vi "Import Project Information From Excel.vi"(0 "Project  path":path=path "C:/Users/L025200.LUXSHARE/Desktop/VNA Aotomatic Data Save Tool 20150327/Project/QSFP+ Project.xls" caption="Project path") -> (16 "Switch Matrix  Name":string, 17 "Report Config":string[](array[string]), 18 "Spec Name":string, 19 "Report Name":string, 20 "S-para Pair Name":string[](array[string])=["TX0", "TX1", "TX2", "TX3", "RX0", "RX1", "RX2", "RX3"], 22 "NEXT Pair Name":string[](array[string])=["TX0-RX0", "TX1-RX0", "TX2-RX0", "TX3-RX0", "TX0-RX1", "TX1-RX1", "TX2-RX1", "TX3-RX1", "TX0-RX2", "TX1-RX2", "TX2-RX2", "TX3-RX2", "TX0-RX3", "TX1-RX3", "TX2-RX3", "TX3-RX3"], 23 "SingleTest Item Name":string[](array[string]), 24 "FEXT Pair Name":string[](array[string])=["TX1-RX0", "TX2-RX0", "TX3-RX0", "TX0-RX1", "TX2-RX1", "TX3-RX1", "TX0-RX2", "TX1-RX2", "TX3-RX2", "TX0-RX3", "TX1-RX3", "TX2-RX3"], 25 "Diff Test Item Name":string[](array[string])=["SDD21", "SDD22", "SCD21", "SCD22", "SCC11", "SCC22", "NEXT", "FEXT"], 26 "Spec Association Col No":string[](array[string])=["1", "2", "NAN", "NAN", "NAN", "NAN", "NAN", "NAN"], 27 "Cal File Path":string[](array[string])=["D:\\CALFILES\\cable.csa"])   [LabVIEW 2011]
panel:
  in  "Excel._Worksheet":refnum<k7>
  in  "Excel._Application":refnum<k7>
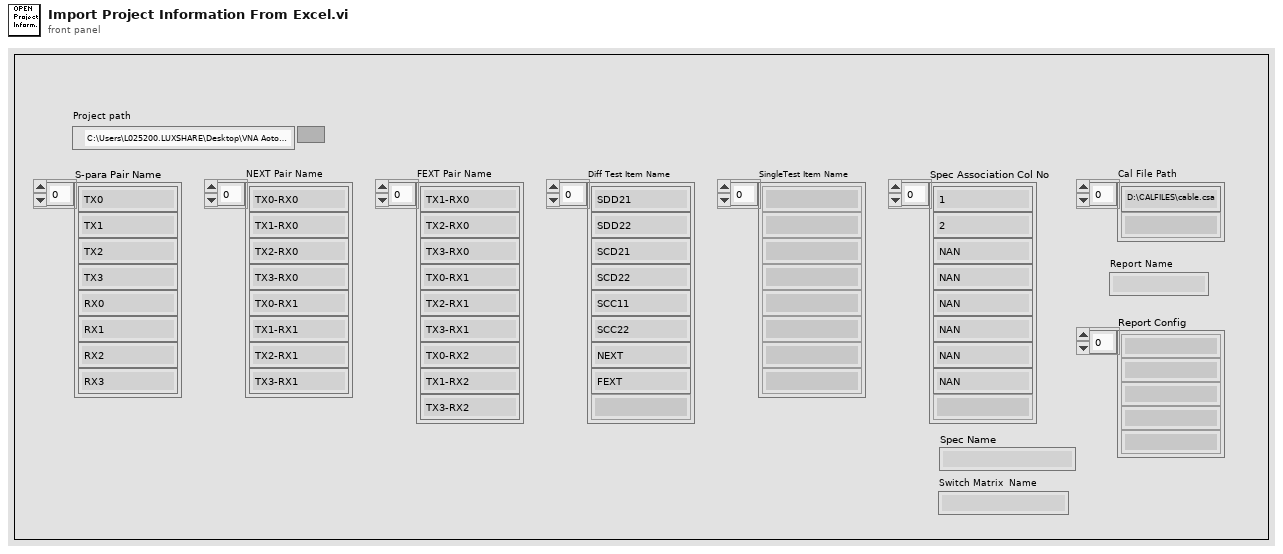
[diagram p1: front panel]
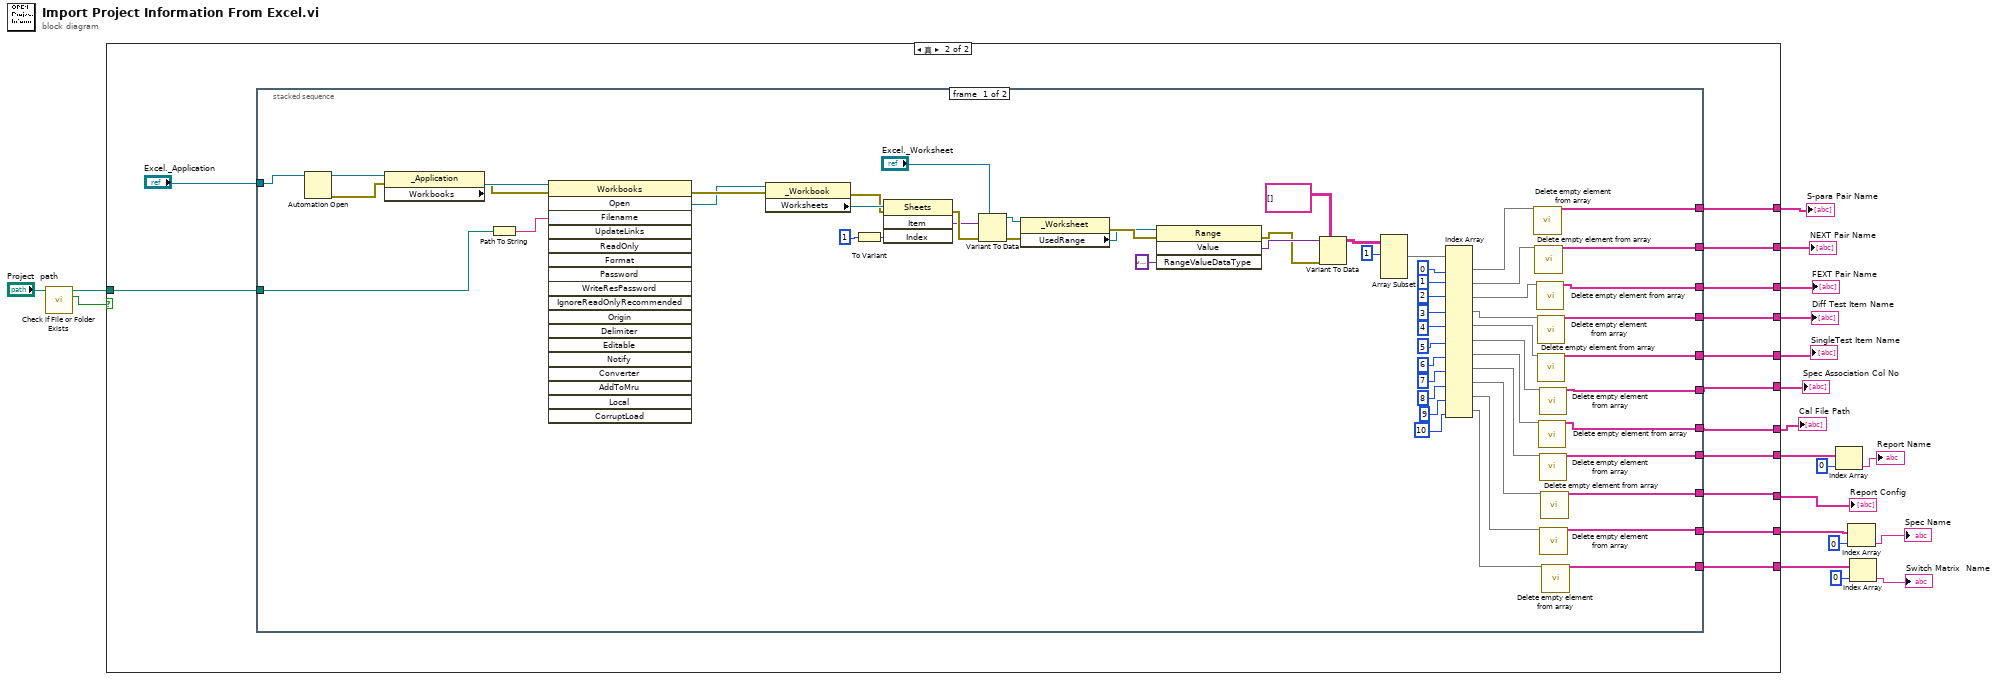
[diagram p0: block diagram]
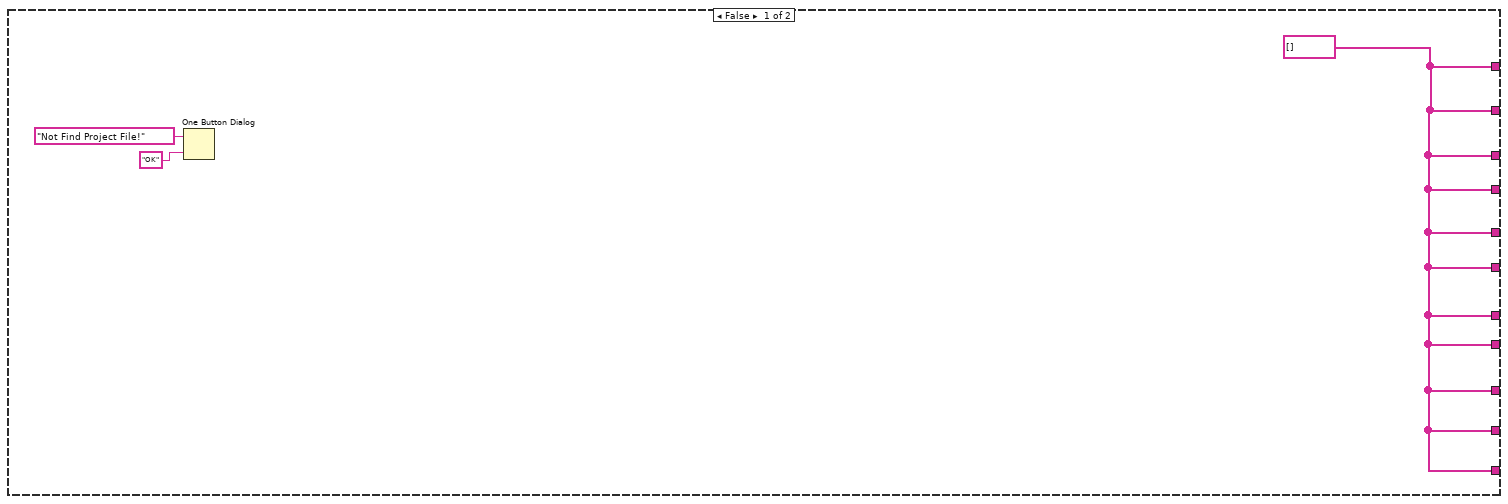
[diagram p2: hidden frame]
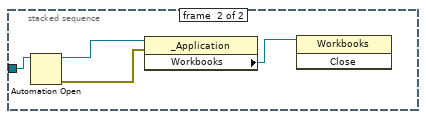
[diagram p3: hidden frame]
diagram:
  n1 = call <vilib>:"Check if File or Folder Exists.vi"("path"="Project  path") -> ("file or folder exists?"=w20:bool, "dup path"=w19:path)  [unwired: 8 in, 1 out]
  n2 = case shown="真" w20 {
    tunnel: w19 -> [_ w35]
    tunnel: [w21 w34] -> w18
    tunnel: [w21 w33] -> w17
    tunnel: [w21 w32] -> w16
    tunnel: [w21 w31] -> w15
    tunnel: [w21 w30] -> w14
    tunnel: [w21 w29] -> w12
    tunnel: [w21 w28] -> w11
    tunnel: [w21 w27] -> w10
    tunnel: [w21 w26] -> w7
    tunnel: [w21 w25] -> w4
    tunnel: [w21 w24] -> w3
    frame False {
      w21 = string[] []
      n3 = One Button Dialog(message="Not Find Project File!" ("消息"), button name ("OK")="OK" ("按钮名称（“确定”）")) -> ()  [unwired: 1 out]
    }
    frame True {
      n4 = stacked-sequence {
        tunnel: "Excel._Application" -> [w61 w98]
        tunnel: w35 -> [w69 _]
        tunnel: [w67 _] -> w34
        tunnel: [w66 _] -> w33
        tunnel: [w65 _] -> w32
        tunnel: [w56 _] -> w30
        tunnel: [w50 _] -> w31
        tunnel: [w51 _] -> w29
        tunnel: [w49 _] -> w28
        tunnel: [w44 _] -> w27
        tunnel: [w43 _] -> w26
        tunnel: [w38 _] -> w25
        tunnel: [w37 _] -> w24
        frame #0 {
          n5 = Automation Open(Automation Refnum=w61) -> (Automation Refnum=w62:refnum<k7>, error out=w96:errorcluster)  [unwired: 3 in]
          n6 = property class="_Application"(reference=w62, error in=w96) -> (error out=w94:errorcluster, "Workbooks"=w95:refnum<k7>)  [unwired: 1 out]
          n7 = Path To String(path=w69) -> (string=w68:string)
          n8 = invoke class="Workbooks" method="Open"(reference=w95, error in=w94, "Filename"=w68) -> (error out=w93:errorcluster, "Open"=w63:refnum<k7>)  [unwired: 15 in, 16 out]
          n9 = property class="_Workbook"(reference=w63, error in=w93) -> (error out=w88:errorcluster, "Worksheets"=w92:refnum<k7>)  [unwired: 1 out]
          n10 = To Variant(anything=1) -> (Variant=w90:variant)
          n11 = invoke class="Sheets" method="Item"(reference=w92, error in=w88, "Index"=w90) -> (error out=w89:errorcluster, "Item"=w87:variant)  [unwired: 1 in, 2 out]
          n12 = Variant To Data(error in=w89, type="Excel._Worksheet", Variant=w87) -> (data=w85:refnum<k7>, error out=w84:errorcluster)
          n13 = property class="_Worksheet"(reference=w85, error in=w84) -> (error out=w81:errorcluster, "UsedRange"=w64:refnum<k7>)  [unwired: 1 out]
          n14 = invoke class="Range" method="Value"(reference=w64, error in=w81, "RangeValueDataType"=variant) -> (error out=w79:errorcluster, "Value"=w83:variant)  [unwired: 1 in, 2 out]
          n15 = Variant To Data(error in=w79, type=string[][] [] ("添加的数组"), Variant=w83) -> (data=w78:string[][])  [unwired: 1 out]
          n16 = Array Subset(array=w78, index (row)=1 ("索引")) -> (w76:string[][])  [unwired: 3 in]
          n17 = Index Array(array=w76, index (col) #1=0 ("禁用的索引 (列)"), index (col) #2=1 ("索引 (列)"), index (col) #3=2 ("索引 (列)"), index (col) #4=3 ("索引 (列)"), index (col) #5=4 ("索引 (列)"), index (col) #6=5 ("索引 (列)"), index (col) #7=6 ("索引 (列)"), index (col) #8=7 ("索引 (列)"), index (col) #9=8 ("索引 (列)"), index (col) #10=9 ("索引 (列)"), index (col) #11=10 ("索引 (列)")) -> (element #1=w72:string[], element #2=w71:string[], element #3=w70:string[], element #4=w58:string[], element #5=w57:string[], element #6=w54:string[], element #7=w52:string[], element #8=w46:string[], element #9=w45:string[], element #10=w40:string[], element #11=w39:string[])  [unwired: 11 in]
          n18 = call "Delete empty element from array.vi"("Array In"=w72) -> ("Array out"=w67:string[])  [unwired: 26 in]
          n19 = call "Delete empty element from array.vi"("Array In"=w71) -> ("Array out"=w66:string[])  [unwired: 26 in]
          n20 = call "Delete empty element from array.vi"("Array In"=w70) -> ("Array out"=w65:string[])  [unwired: 26 in]
          n21 = call "Delete empty element from array.vi"("Array In"=w58) -> ("Array out"=w56:string[])  [unwired: 26 in]
          n22 = call "Delete empty element from array.vi"("Array In"=w57) -> ("Array out"=w49:string[])  [unwired: 26 in]
          n23 = call "Delete empty element from array.vi"("Array In"=w52) -> ("Array out"=w51:string[])  [unwired: 26 in]
          n24 = call "Delete empty element from array.vi"("Array In"=w54) -> ("Array out"=w50:string[])  [unwired: 26 in]
          n25 = call "Delete empty element from array.vi"("Array In"=w46) -> ("Array out"=w44:string[])  [unwired: 26 in]
          n26 = call "Delete empty element from array.vi"("Array In"=w40) -> ("Array out"=w38:string[])  [unwired: 26 in]
          n27 = call "Delete empty element from array.vi"("Array In"=w45) -> ("Array out"=w43:string[])  [unwired: 26 in]
          n28 = call "Delete empty element from array.vi"("Array In"=w39) -> ("Array out"=w37:string[])  [unwired: 26 in]
        }
        frame #1 {
          n29 = Automation Open(Automation Refnum=w98) -> (Automation Refnum=w99:refnum<k7>, error out=w100:errorcluster)  [unwired: 3 in]
          n30 = property class="_Application"(reference=w99, error in=w100) -> ("Workbooks"=w97:refnum<k7>)  [unwired: 2 out]
          n31 = invoke class="Workbooks" method="Close"(reference=w97) -> ()  [unwired: 2 in, 3 out]
        }
      }
    }
  }
  "S-para Pair Name" <- w18
  "NEXT Pair Name" <- w17
  "FEXT Pair Name" <- w16
  "Spec Association Col No" <- w15
  "Diff Test Item Name" <- w14
  "Cal File Path" <- w12
  "SingleTest Item Name" <- w11
  "Report Config" <- w7
  n32 = Index Array(array=w10, index=0 ("索引")) -> (element=→"Report Name":string)
  n33 = Index Array(array=w4, index=0 ("索引")) -> (element=→"Spec Name":string)
  n34 = Index Array(array=w3, index=0 ("索引")) -> (element=→"Switch Matrix  Name":string)
